vi "IDE_Example.vi"() -> ()   [LabVIEW 2020]
uses:
  Subs/ColorText/Code.xctl
  Subs/Console XCtrl/Console_Xctrl.xctl
  Subs/Server XCtrl/Server.xctl
panel:
  in  "Clean":bool
  in  "PC Save":bool
  in  "PC path":path
  in  "Files":bool
  in  "Server":bool
  in  "Help":bool
  in  "Server":path(xcontrol)=path "/Users/crogers/GitHub/Summer2020/LabVIEWCode/Servers/Jens.vi"
  out "REPL":string(xcontrol)
  in  "Clear":bool
  in  "Save":bool
  in  "Stop":bool
  in  "Run":bool
  in  "Name":string="code.py"
  in  "Code":string(xcontrol)="import os\n\nfor i in range(10):\n     print(i)\n"
  # "¨Processor"
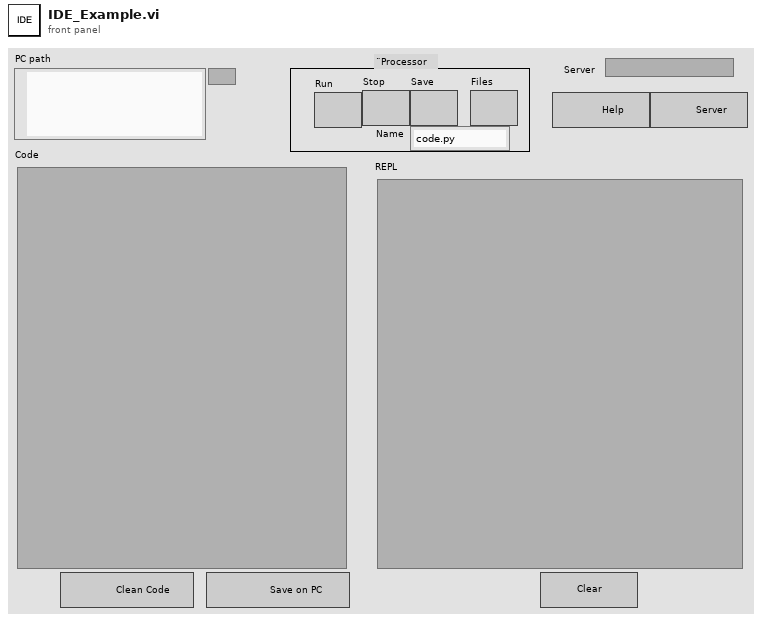
[diagram p1: front panel]
types:
  T1 = cluster{"Quote":u32, "Comment":u32, "Python":u32, "Text":u32, "Triple Quote":u32, "function":u32, "Line numbers":u32, "REPL Err":u32, "REPL Text":u32, "Text Bkgd":u32, "REPL Bkgd":u32}
  T2 = enum8{"Enabled", "Disabled", "Disabled and Grayed Out"}
  T3 = typedef "eventvkey.ctl" = enum16{"ASCII", "Enter", "Return", "Shift", "Ctrl", "Alt", "Cmd", "Opt", "Caps", "NumLock", "Clear", "Break", "Up", "Down", "Left", "Right", "Insert", "Delete", "Home", "End", "PageUp", "PageDown", "Escape", "Help", "Pause", "ScrollLock", "F1", "F2", "F3", "F4", "F5", "F6", "F7", "F8", "F9", "F10", "F11", "F12", "F13", "F14", "F15", "F16", "F17", "F18", "F19", "F20", "F21", "F22", "F23", "F24", "Play", "VolumeUp", "VolumeDown", "Mute", "Two Byte Char"}
  T4 = cluster{"Shift":bool, "Ctrl":bool, "Alt":bool, "Cmd":bool, "Opt":bool}
  T5 = cluster{"Char":i16, "VKey":T3, "PlatMods":cluster{"Shift":bool, "Ctrl":bool, "Alt":bool, "Cmd":bool, "Opt":bool}}
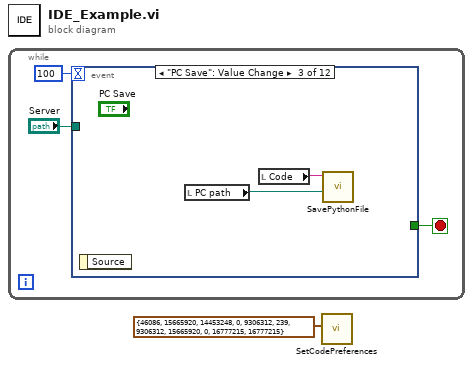
[diagram p0: block diagram]
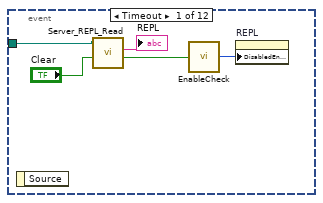
[diagram p2: hidden frame]
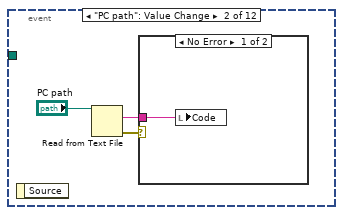
[diagram p3: hidden frame]
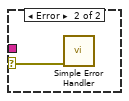
[diagram p4: hidden frame]
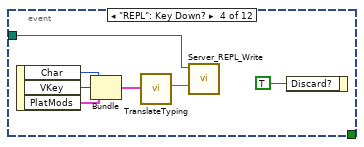
[diagram p5: hidden frame]
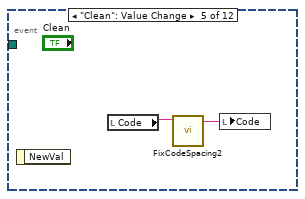
[diagram p6: hidden frame]
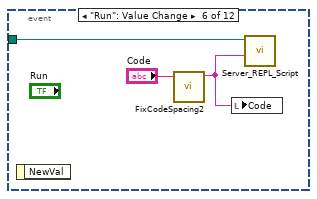
[diagram p7: hidden frame]
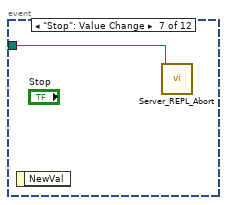
[diagram p8: hidden frame]
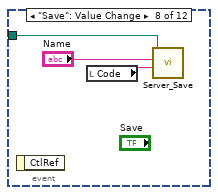
[diagram p9: hidden frame]
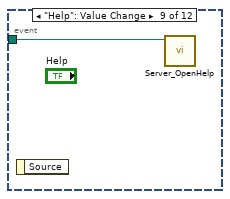
[diagram p10: hidden frame]
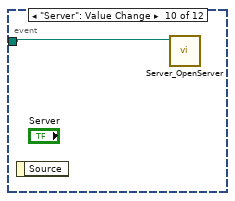
[diagram p11: hidden frame]
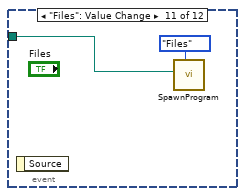
[diagram p12: hidden frame]
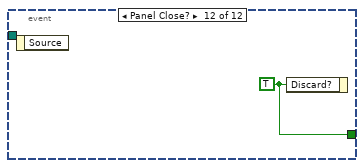
[diagram p13: hidden frame]
diagram:
  n1 = while {
    stop <- w3 stop-if-true
    n2 = event shown="[2] \"PC Save\": Value Change" {
      selector: _ -> [_ _ _ _ _ _ _ _ _ _ _ _]
      dyn-events: _ -> [_ _ _ _ _ _ _ _ _ _ _ _]
      timeout: 100 -> [_ _ _ _ _ _ _ _ _ _ _ _]
      tunnel: [_ _ _ _ _ _ _ _ _ _ _ w37] -> w3
      tunnel: "Server" -> [w7 _ _ w17 _ w27 w29 w30 w33 w34 w36 _]
      event Timeout {
        n3 = event-data() -> ()  [unwired: 1 in, 1 out]
        n4 = call "Server_REPL_Read.vi"("Clear"="Clear", "Server"=w7) -> ("Running?"=w8:bool, "REPL"=→"REPL":string)  [unwired: 7 in, 1 out]
        n5 = call "EnableCheck.vi"("Enable?"=w8) -> ("Enum"=w9:T2)
        n6 = property on="REPL" class="Console_Xctrl (strict)"("DisabledEnum"=w9) -> ()  [unwired: 2 in, 2 out]
      }
      event "PC path": Value Change {
        n7 = event-data() -> ()  [unwired: 1 in, 1 out]
        n8 = Read from Text File(file (use dialog)="PC path") -> (text=w11:string, error out=w12:errorcluster)  [unwired: 3 in, 2 out]
        n9 = case shown="No Error" w12 {
          selector: w12 -> [_ w14]
          tunnel: w11 -> [w13 _]
          frame No Error {
            n10 = local write "Code"(w13) -> ()
          }
          frame Error {
            n11 = call <vilib>:"Simple Error Handler.vi"("error in (no error)"=w14) -> ()  [unwired: 4 in, 5 out]
          }
        }
      }
      event "PC Save": Value Change {
        n12 = event-data() -> ()  [unwired: 1 in, 1 out]
        n13 = local read "PC path"() -> (w15:path)
        n14 = local read "Code"() -> (w16:string)
        n15 = call "SavePythonFile.vi"("path"=w15, "Code"=w16) -> ()  [unwired: 10 in]
      }
      event "REPL": Key Down? {
        n16 = event-data() -> ("Char"=w22:i16, "VKey"=w21:T3, "PlatMods"=w19:T4)  [unwired: 1 in]
        n17 = Bundle("Char"=w22, "VKey"=w21, "PlatMods"=w19) -> (w23:T5)  [unwired: 1 in]
        n18 = call "TranslateTyping.vi"("Cluster"=w23) -> ("key"=w18:string)  [unwired: 10 in]
        n19 = call "Server_REPL_Write.vi"("Code"=w18, "Server"=w17) -> ()  [unwired: 9 in, 1 out]
        n20 = event-data("Discard?"=TRUE) -> ()  [unwired: 1 in, 1 out]
      }
      event "Clean": Value Change {
        n21 = event-data() -> ()  [unwired: 1 in, 1 out]
        n22 = local read "Code"() -> (w24:string)
        n23 = call "FixCodeSpacing2.vi"("Code"=w24) -> ("Cleaned"=w25:string)  [unwired: 10 in]
        n24 = local write "Code"(w25) -> ()
      }
      event "Run": Value Change {
        n25 = event-data() -> ()  [unwired: 1 in, 1 out]
        n26 = call "FixCodeSpacing2.vi"("Code"="Code") -> ("Cleaned"=w26:string)  [unwired: 10 in]
        n27 = local write "Code"(w26) -> ()
        n28 = call "Server_REPL_Script.vi"("Code"=w26, "Server"=w27) -> ()  [unwired: 9 in, 1 out]
      }
      event "Stop": Value Change {
        n29 = event-data() -> ()  [unwired: 1 in, 1 out]
        n30 = call "Server_REPL_Abort.vi"("Server"=w29) -> ()  [unwired: 10 in, 1 out]
      }
      event "Save": Value Change {
        n31 = event-data() -> ()  [unwired: 1 in, 1 out]
        n32 = local read "Code"() -> (w32:string)
        n33 = call "Server_Save.vi"("Code"=w32, "Name"="Name", "Server"=w30) -> ()  [unwired: 8 in, 1 out]
      }
      event "Help": Value Change {
        n34 = event-data() -> ()  [unwired: 1 in, 1 out]
        n35 = call "Server_OpenHelp.vi"("Server"=w33) -> ()  [unwired: 10 in, 1 out]
      }
      event "Server": Value Change {
        n36 = event-data() -> ()  [unwired: 1 in, 1 out]
        n37 = call "Server_OpenServer.vi"("Server"=w34) -> ()  [unwired: 10 in, 1 out]
      }
      event "Files": Value Change {
        n38 = event-data() -> ()  [unwired: 1 in, 1 out]
        n39 = call "SpawnProgram.vi"("Server"=w36, "Dialog"=enum16{"Help", "Files"}."Files") -> ()  [unwired: 10 in]
      }
      event Panel Close? {
        w37 = TRUE ("Discard?")
        n40 = event-data() -> ()  [unwired: 1 in, 1 out]
        n41 = event-data("Discard?"=w37) -> ()  [unwired: 1 in, 1 out]
      }
    }
  }
  n42 = call "SetCodePreferences.vi"("Color choices"=T1 {"Quote"=46086, "Comment"=15665920, "Python"=14453248, "Text"=0, "Triple Quote"=9306312, "function"=239, "Line numbers"=9306312, "REPL Err"=15665920, "REPL Text"=0, "Text Bkgd"=16777215, "REPL Bkgd"=16777215}) -> ()  [unwired: 11 in]
